vi "SR830_highfreq_readout.vi"(0 "address string":string="30", 1 "X channel":tag="Dev2/ai0", 5 "number of samples per channel":i32=50000, 7 "sample mode":i32(ring)=10178 items=["Finite Samples"=10178, "Continuous Samples"=10123], 9 "rate":dbl=5000.0 format="%0.2f", 11 "error in (no error)":errorcluster, 12 "Y channel":tag="Dev2/ai1", 13 "Dc Voltage (V)":dbl=1.0 format="%0.2f") -> (2 "Lock In Signal Spectrum (mV/V) X,Y,R":cluster{"f0":dbl, "df":dbl, "magnitude":dbl[]}[](graph), 3 "Lockin R (mV/V)":waveform(dbl)(graph), 4 "Lock In Signal Spectrum (mV/V)":cluster{"f0":dbl, "df":dbl, "magnitude":dbl[]}(graph), 6 "R":dbl[](graph), 8 "Lockin X,Y,R (mV/V)":waveform(dbl)[](graph), 10 "Theta":dbl[](graph), 14 "Lockin Theta":waveform(dbl)(graph), 15 "error out":errorcluster)   [LabVIEW 2013]
uses:
  <vilib>/DAQmx/read.llb/DAQmx Read (Analog 2D DBL NChan NSamp).vi
  <vilib>/DAQmx/create/channels.llb/DAQmx Create Channel (AI-Voltage-Basic).vi
  <vilib>/DAQmx/configure/timing.llb/DAQmx Timing (Sample Clock).vi
  <vilib>/DAQmx/miscellaneous.llb/DAQmx Fill In Error Info.vi
  <vilib>/express/express analysis/Spectral/Block/exnSpectralBlock spectral measurements peak poly.vi
  <vilib>/express/express analysis/Spectral/Block/exnSpectralBlock spectral measurements peak array WFM.vi
  <vilib>/express/express analysis/Spectral/Block/exnSpectralBlock spectral measurements peak WFM.vi
  <vilib>/express/express analysis/Spectral/XNode/ExpressSpectralMeasurementsBlockNode.xnode
  <resource>/objmgr/daqmx.rc
panel:
  out "Y":dbl[](array[numeric])
  out "X":dbl[](array[numeric])
  in  "minimum value":dbl=-10.0 format="%0.2f"
  in  "maximum value":dbl=10.0 format="%0.2f"
  in  "stop":bool
  out "Sensitivity":dbl
  in  "Tab Control":enum32{"Page 1", "Spectrum", "Page 2"}(tab)
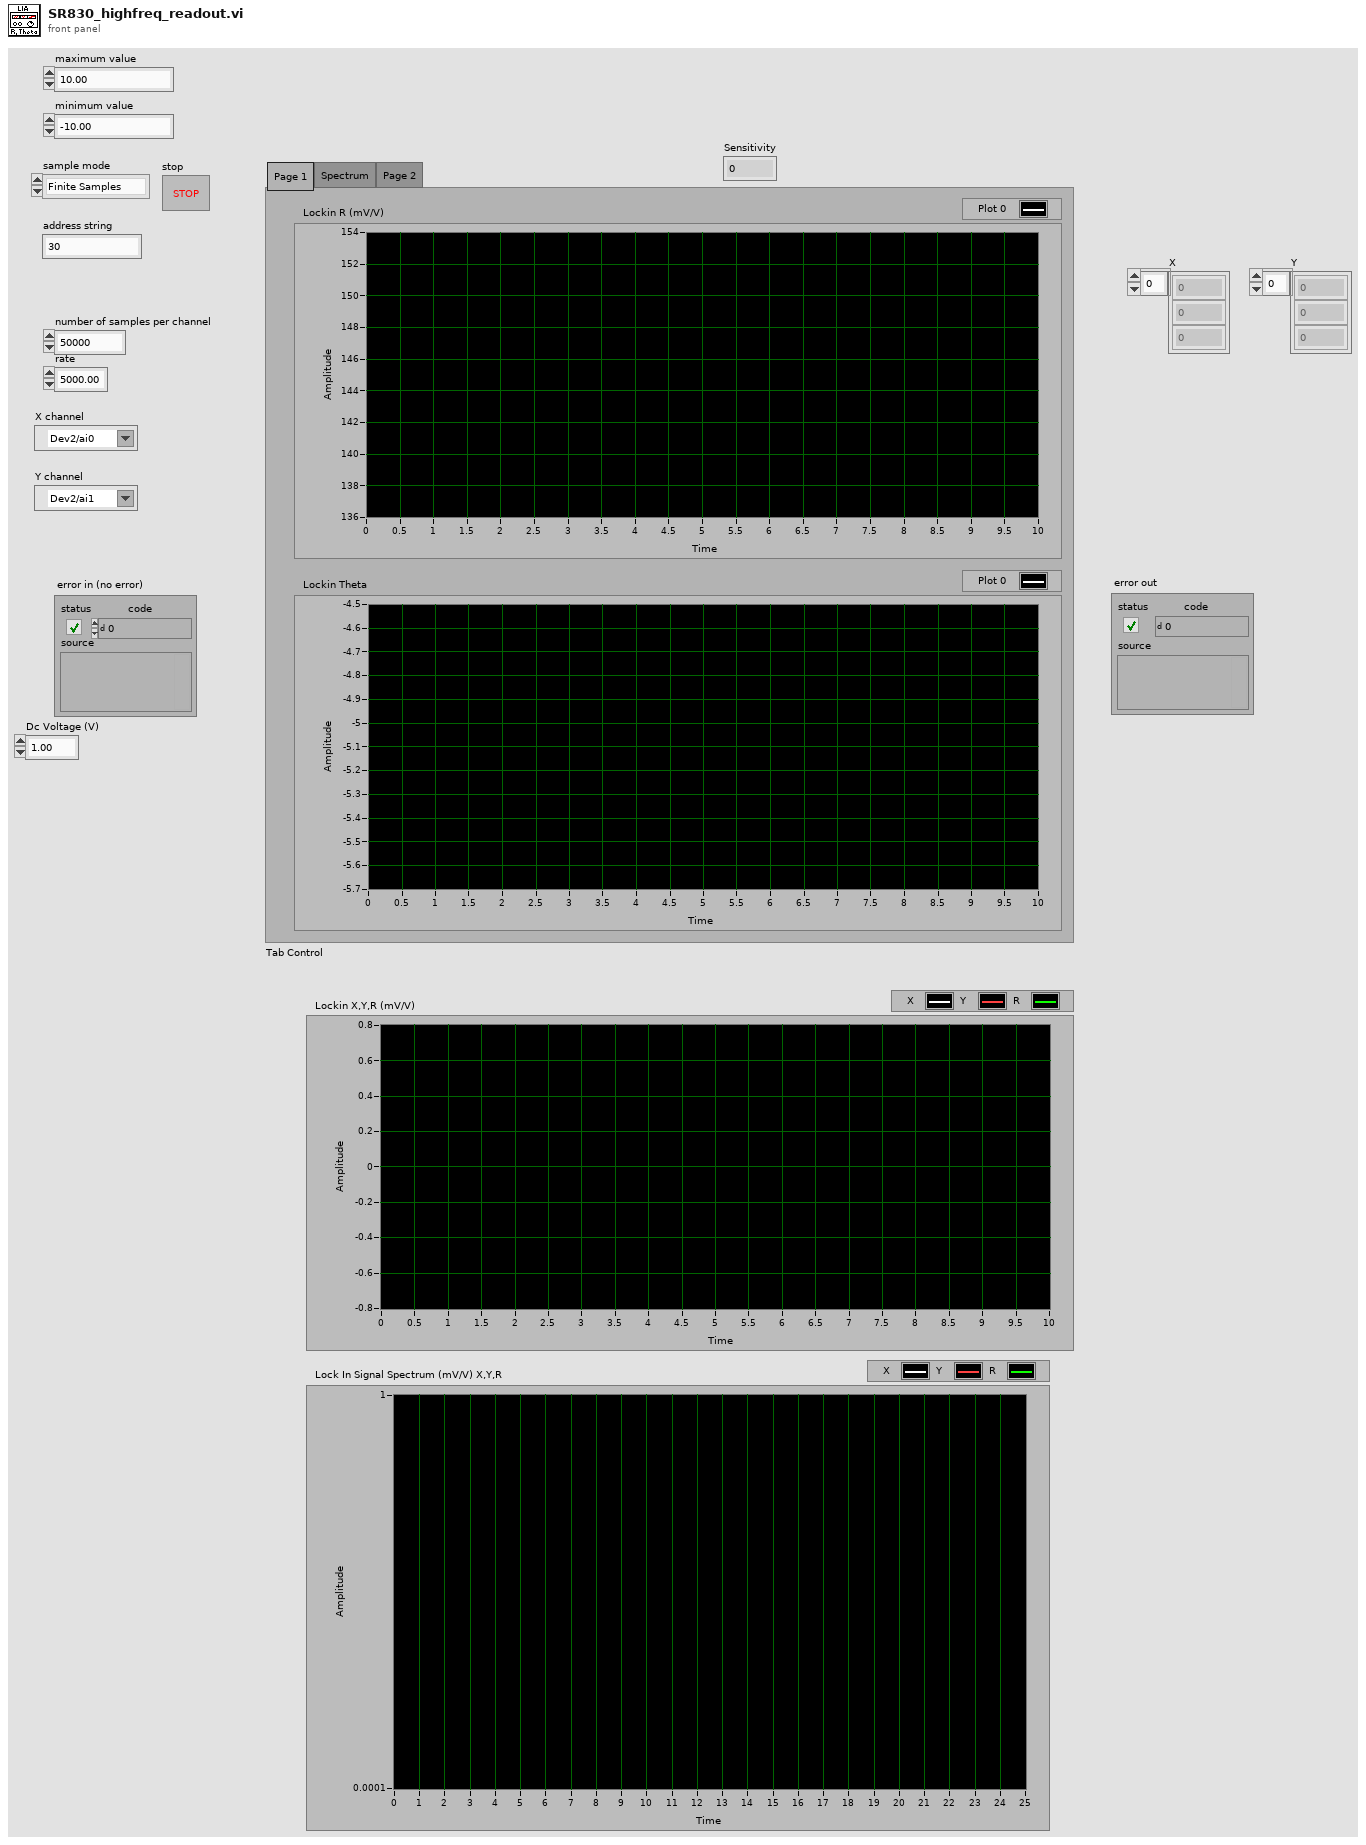
[diagram p1: front panel]
types:
  T1 = cluster{"averaging mode":u16, "weighting mode":u16, "number of averages":u32}
  T2 = cluster{"dB On (F)":bool, "unwrap phase (F)":bool, "convert to degree (F)":bool}
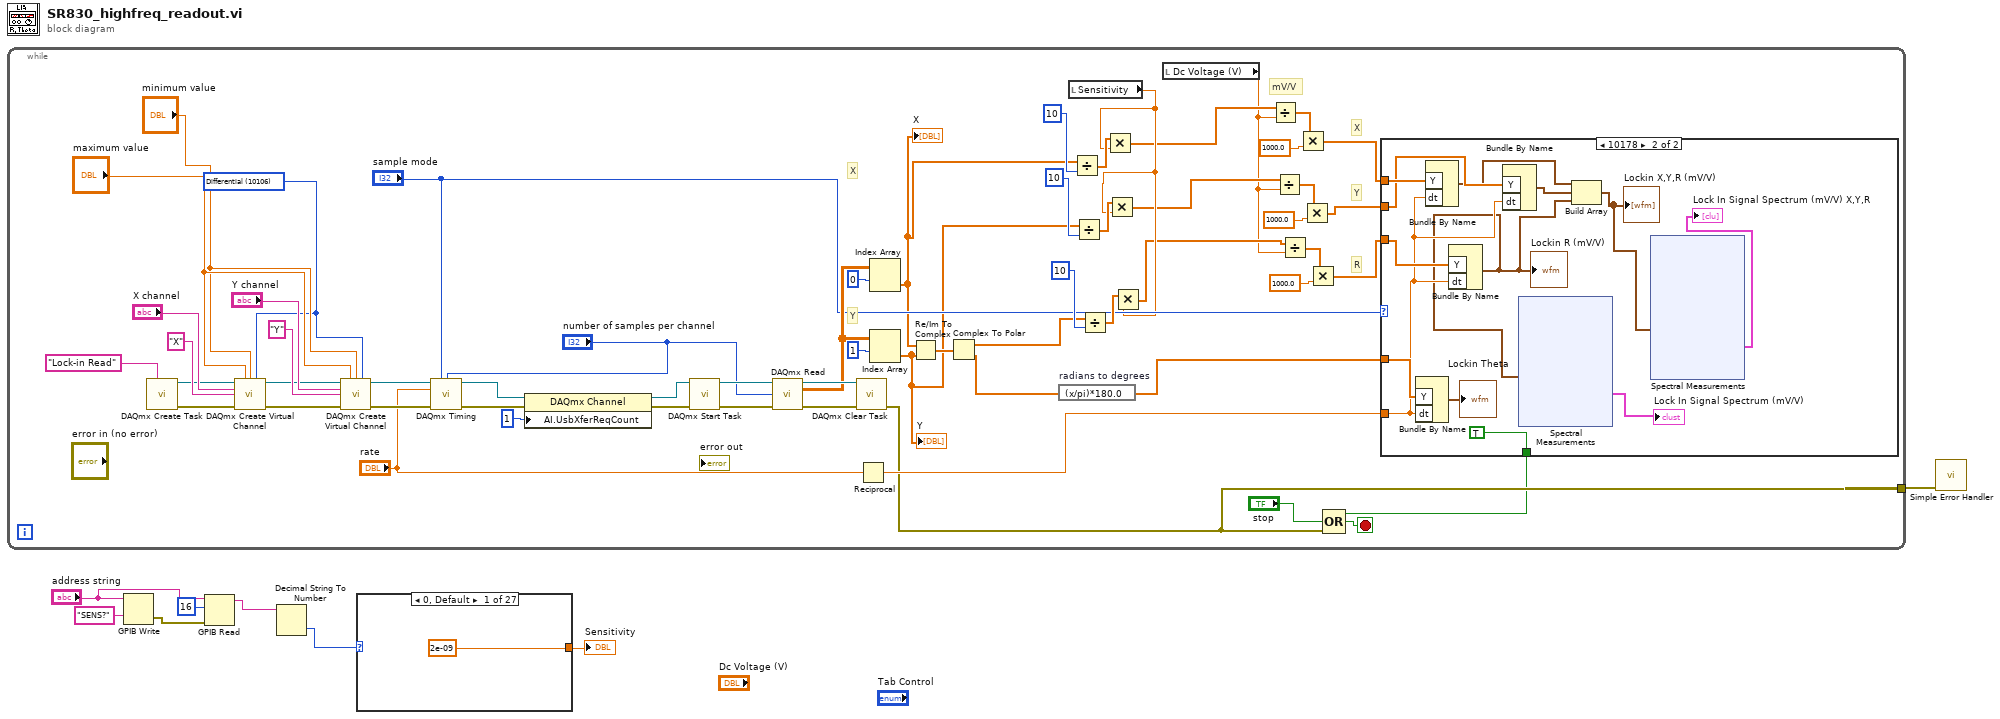
[diagram p0: block diagram]
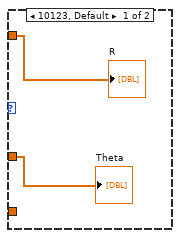
[diagram p2: hidden frame]
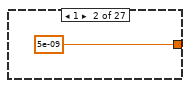
[diagram p3: hidden frame]
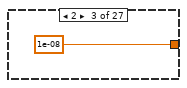
[diagram p4: hidden frame]
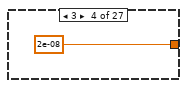
[diagram p5: hidden frame]
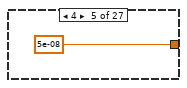
[diagram p6: hidden frame]
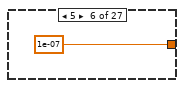
[diagram p7: hidden frame]
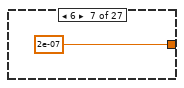
[diagram p8: hidden frame]
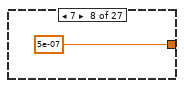
[diagram p9: hidden frame]
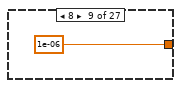
[diagram p10: hidden frame]
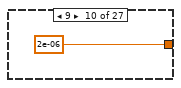
[diagram p11: hidden frame]
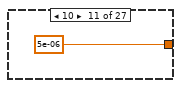
[diagram p12: hidden frame]
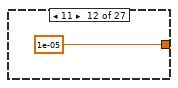
[diagram p13: hidden frame]
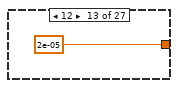
[diagram p14: hidden frame]
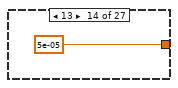
[diagram p15: hidden frame]
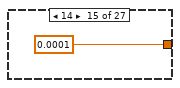
[diagram p16: hidden frame]
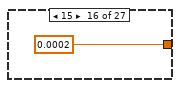
[diagram p17: hidden frame]
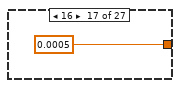
[diagram p18: hidden frame]
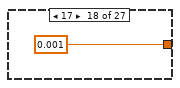
[diagram p19: hidden frame]
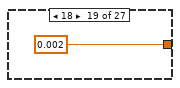
[diagram p20: hidden frame]
diagram:
  n1 = while {
    tunnel: [w35] -> w1
    stop <- w36 stop-if-true
    w9 = 10106 items=["default"=-1, "RSE"=10083, "NRSE"=10078, "Differential"=10106, "Pseudodifferential"=12529] ("input terminal configuration")
    # "mV/V"
    # "R"
    # "Y"
    # "X"
    # "Y"
    # "X"
    n2 = call <vilib>:"DAQmx Create Task.vi"("new task name"="Lock-in Read") -> ("task out"=w58:refnum<k21>, "error out"=w57:errorcluster)  [unwired: 13 in]
    n3 = call-poly <vilib>:"DAQmx Create Virtual Channel.vi"("task in"=w58, "maximum value"="maximum value", "minimum value"="minimum value", "input terminal configuration"=w9, "physical channels"="X channel", "name to assign"="X", "error in"=w57) -> ("task out"=w59:refnum<k21>, "error out"=w60:errorcluster)  [unwired: 7 in]
    n4 = call-poly <vilib>:"DAQmx Create Virtual Channel.vi"("task in"=w59, "maximum value"="maximum value", "minimum value"="minimum value", "input terminal configuration"=w9, "physical channels"="Y channel", "name to assign"="Y", "error in"=w60) -> ("task out"=w67:refnum<k21>, "error out"=w68:errorcluster)  [unwired: 7 in]
    n5 = call-poly <vilib>:"DAQmx Timing.vi"("task/channels in"=w67, "sample mode"="sample mode", "samples per channel"="number of samples per channel", "rate"="rate", "error in"=w68) -> ("task out"=w53:refnum<k21>, "error out"=w55:errorcluster)  [unwired: 9 in]
    n6 = property class="DAQmx Channel"(reference=w53, error in=w55, "AI.UsbXferReqCount"=u32 1) -> (reference out=w52:refnum<k21>, error out=w54:errorcluster)
    n7 = call <vilib>:"DAQmx Start Task.vi"("task/channels in"=w52, "error in"=w54) -> ("task out"=w65:refnum<k21>, "error out"=w66:errorcluster)  [unwired: 12 in]
    n8 = call-poly <vilib>:"DAQmx Read.vi"("task/channels in"=w65, "number of samples per channel"="number of samples per channel", "error in"=w66) -> ("task out"=w49:refnum<k21>, "data"=w47:dbl[][], "error out"=w50:errorcluster)  [unwired: 10 in]
    n9 = call <vilib>:"DAQmx Clear Task.vi"("task in"=w49, "error in"=w50) -> ("error out"=w35:errorcluster)  [unwired: 13 in]
    n10 = Reciprocal(x="rate") -> (1/x=w43:dbl)
    n11 = Index Array(array=w47, index (row)=0) -> (element=w25:dbl[])  [unwired: 1 in]
    "X" <- w25
    n12 = Index Array(array=w47, index (row)=1) -> (element=w24:dbl[])  [unwired: 1 in]
    "Y" <- w24
    n13 = Re/Im To Complex(1:w24, 2:w25) -> (0:w45:cdb[])
    n14 = Complex To Polar(r * e^(i*theta)=w45) -> (r=w30:dbl[], theta=w42:dbl[])
    n15 = expression code="(x/pi)*180.0" "radians to degrees"(w42) -> (w41:dbl[])
    n16 = local read "Sensitivity"() -> (w23:dbl)
    n17 = Divide(x=w25, y=10 ("Waveform")) -> (x/y=w26:dbl[])
    n18 = Divide(x=w24, y=10 ("Waveform")) -> (x/y=w29:dbl[])
    n19 = Divide(x=w30, y=10 ("Waveform")) -> (x/y=w38:dbl[])
    n20 = Multiply(x=w26, y=w23) -> (x*y=w21:dbl[])
    n21 = Multiply(x=w29, y=w23) -> (x*y=w16:dbl[])
    n22 = Multiply(x=w38, y=w23) -> (x*y=w12:dbl[])
    n23 = local read "Dc Voltage (V)"() -> (w10:dbl)
    n24 = Divide(x=w21, y=w10) -> (x/y=w20:dbl[])
    n25 = Divide(x=w16, y=w10) -> (x/y=w18:dbl[])
    n26 = Divide(x=w12, y=w10) -> (x/y=w13:dbl[])
    n27 = Multiply(x=w20, y=1000.0 ("rate")) -> (x*y=w19:dbl[])
    n28 = Multiply(x=w18, y=1000.0 ("rate")) -> (x*y=w15:dbl[])
    n29 = Multiply(x=w13, y=1000.0 ("rate")) -> (x*y=w11:dbl[])
    n30 = case shown="10178" "sample mode" {
      tunnel: w43 -> [_ w76]
      tunnel: w41 -> [w70 w80]
      tunnel: w11 -> [w69 w79]
      tunnel: [_ TRUE ("value")] -> w31
      tunnel: w19 -> [_ w78]
      tunnel: w15 -> [_ w77]
      frame 10123, Default {
        "R" <- w69
        "Theta" <- w70
      }
      frame 10178 {
        n31 = Bundle By Name("Y"=w80, "dt"=w76) -> (→"Lockin Theta":waveform(dbl))  [unwired: 1 in]
        n32 = Bundle By Name("Y"=w78, "dt"=w76) -> (w75:waveform(dbl))  [unwired: 1 in]
        n33 = Bundle By Name("Y"=w79, "dt"=w76) -> (w73:waveform(dbl))  [unwired: 1 in]
        "Lockin R (mV/V)" <- w73
        n34 = Bundle By Name("Y"=w77, "dt"=w76) -> (w74:waveform(dbl))  [unwired: 1 in]
        n35 = xnode "Spectral Measurements"("Signals"=w73) -> ("FFT - (Peak)"=→"Lock In Signal Spectrum (mV/V)":cluster{"f0":dbl, "df":dbl, "magnitude":dbl[]})  [unwired: 1 in, 2 out]
        n36 = Build Array(w75, w74, w73) -> (w72:waveform(dbl)[])
        "Lockin X,Y,R (mV/V)" <- w72
        n37 = xnode "Spectral Measurements"("Signals"=w72) -> ("FFT - (Peak)"=→"Lock In Signal Spectrum (mV/V) X,Y,R":cluster{"f0":dbl, "df":dbl, "magnitude":dbl[]}[])  [unwired: 1 in, 2 out]
      }
    }
    n38 = Compound Arithmetic op=OR(w31, "stop", w35) -> (w36:bool)
  }
  n39 = GPIB Write(0:"address string", 1:"SENS?" ("data")) -> (6:w7:errorcluster)  [unwired: 3 in, 1 out]
  n40 = GPIB Read(0:"address string", 1:16 ("byte count"), 3:w7) -> (5:w5:string)  [unwired: 2 in, 2 out]
  n41 = Decimal String To Number(string=w5) -> (number=w3:i32)  [unwired: 2 in, 1 out]
  n42 = case shown="0, Default" w3 {
    tunnel: [2e-09 5e-09 1e-08 2e-08 5e-08 1e-07 2e-07 5e-07 1e-06 2e-06 5e-06 1e-05 2e-05 5e-05 0.0001 0.0002 0.0005 0.001 0.002 0.005 0.01 0.02 0.05 0.1 0.2 0.5 1] -> w2
    frame 0, Default {
    }
    frame 1 {
    }
    frame 2 {
    }
    frame 3 {
    }
    frame 4 {
    }
    frame 5 {
    }
    frame 6 {
    }
    frame 7 {
    }
    frame 8 {
    }
    frame 9 {
    }
    frame 10 {
    }
    frame 11 {
    }
    frame 12 {
    }
    frame 13 {
    }
    frame 14 {
    }
    frame 15 {
    }
    frame 16 {
    }
    frame 17 {
    }
    frame 18 {
    }
    frame 19 {
    }
    frame 20 {
    }
    frame 21 {
    }
    frame 22 {
    }
    frame 23 {
    }
    frame 24 {
    }
    frame 25 {
    }
    frame 26 {
    }
  }
  "Sensitivity" <- w2
  n43 = call <vilib>:"Simple Error Handler.vi"("error in (no error)"=w1) -> ()  [unwired: 4 in, 5 out]
